vi "counter.vi"(0 "mode":enum16{"increment", "decrement", "reset"}(ring), 5 "add":i32=1, 7 "limit":i32=100, 11 "error in (no error)":errorcluster) -> (4 "limit reached?":bool, 15 "error out":errorcluster)   [LabVIEW 2019, in "Service.lvlib"]
uses:
  Service.lvlib
panel:
  out "counter value":i32
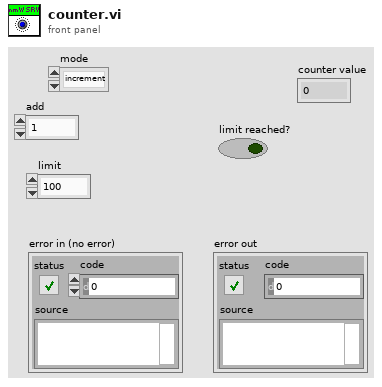
[diagram p1: front panel]
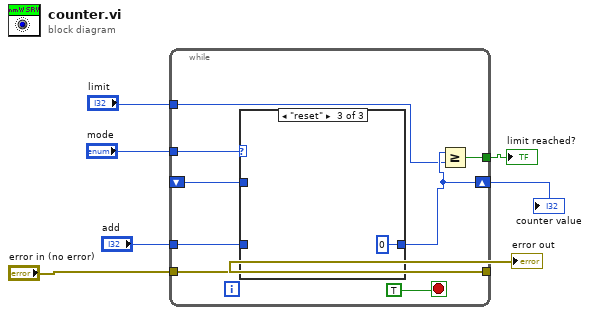
[diagram p0: block diagram]
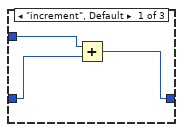
[diagram p2: hidden frame]
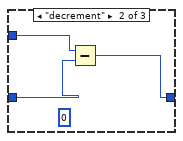
[diagram p3: hidden frame]
diagram:
  n1 = while {
    tunnel: "error in (no error)" -> [w15]
    tunnel: [w15] -> w5
    tunnel: "mode" -> [w14]
    tunnel: "add" -> [w13]
    shift-right: [w11] -> w1
    shift-left: _ -> [w8]
    tunnel: [w9] -> w3
    tunnel: "limit" -> [w10]
    stop <- TRUE stop-if-true
    n2 = case shown="\"reset\"" w14 {
      tunnel: w13 -> [w17 w20 _]
      tunnel: [w16 w19 0] -> w11
      tunnel: w8 -> [w18 w21 _]
      frame "increment", Default {
        n3 = Add(x=w18, y=w17) -> (x+y=w16:i32)
      }
      frame "decrement" {
        (unwired) 0 ("add")
        n4 = Subtract(x=w21, y=w20) -> (x-y=w19:i32)
      }
      frame "reset" {
      }
    }
    n5 = Greater Or Equal?(x=w11, y=w10) -> (x >= y?=w9:bool)
  }
  "limit reached?" <- w3
  "error out" <- w5
  "counter value" <- w1
